vi "Read Server Refnum.vi"(8 "error in (no error)":errorcluster, 11 "OPC UA runtime in":refnum<class "OPC UA Server runtime.lvclass">) -> (0 "error out":errorcluster, 2 "Server Refnum":refnum<k21>, 3 "OPC UA runtime out":refnum<class "OPC UA Server runtime.lvclass">)   [LabVIEW 2013, in "OPC UA Server runtime.lvclass"]
uses:
  OPC UA Server runtime.lvclass
  OPC UA Server runtime.lvclass/OPC UA Server runtime.ctl
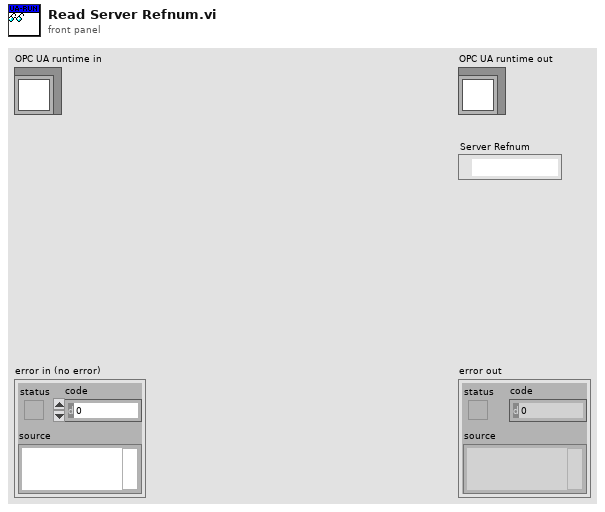
[diagram p1: front panel]
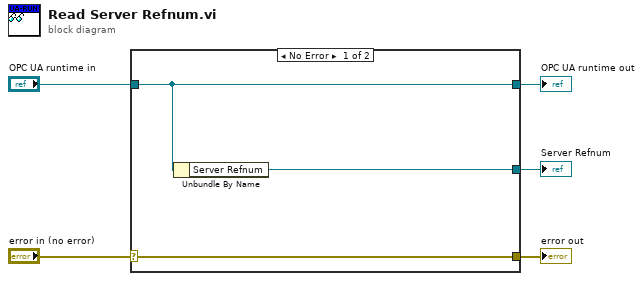
[diagram p0: block diagram]
diagram:
  n1 = case shown="No Error" "error in (no error)" {
    selector: "error in (no error)" -> [w8 w9]
    tunnel: [w8 w9] -> w4
    tunnel: [w7 w10] -> w2
    tunnel: "OPC UA runtime in" -> [w7 w10]
    tunnel: [w6 _] -> w1
    frame No Error {
      n2 = Unbundle By Name(w7) -> ("Server Refnum"=w6:refnum<k21>)
    }
    frame Error {
    }
  }
  "error out" <- w4
  "OPC UA runtime out" <- w2
  "Server Refnum" <- w1
